vi "Read Config Settings from INI file.vi"(1 "Hardware Configuration":T1={"SEM X coil"="SEM-X", "SEM Y coil"="SEM-Y", "FIB X coil"="FIB/ao0", "FIB Y coil"="FIB/ao1", "FIB Detector"="FIB/ai1", "SEM Detectors"="Detectors", "Det min (V)"=-10.0, "Det max (V)"=10.0, "Eanable COM"=TRUE, "COM port"="COM1", "FIB Beam blank"="FIB/port0/line0", "FIB Ext Scan"="FIB/port0/line1", "Det. FIB-NI auto switch"="FIB/port0/line2", "Post #1up"="Log/ao0", "Post #1down"="Log/ao1", "Post #2up"="Log/ao2", "Post #2down"="Log/ao3", "Machine Type"=2, "FIB Faraday Cup"="FIB/ai3", "Configuration file"=path "D:/3D FIB-SEM Files/Feiss.ini", "SEM Max FOV (um)"=350.0, "Machine ID"="Jeiss6/Merlin-xxxx", "Save config file"=FALSE, "Temperature port"="COM3", "Brightness A"=35.0, "Contrast A"=28.0, "Detector B name"="ESB @ 600 V", "Brightness B"=30.0, "Contrast B"=38.0, "Logging Device"="Log"} {"Machine Type" items=["Feiss", "NVision", "Jeiss"]}) -> (8 "Hardware Configuration Out":T1={"SEM X coil"="SEM-X", "SEM Y coil"="SEM-Y", "FIB X coil"="FIB/ao0", "FIB Y coil"="FIB/ao1", "FIB Detector"="FIB/ai1", "SEM Detectors"="Detectors", "Det min (V)"=-10.0, "Det max (V)"=10.0, "Eanable COM"=TRUE, "COM port"="COM1", "FIB Beam blank"="FIB/port0/line0", "FIB Ext Scan"="FIB/port0/line1", "Det. FIB-NI auto switch"="FIB/port0/line2", "Post #1up"="Log/ao0", "Post #1down"="Log/ao1", "Post #2up"="Log/ao2", "Post #2down"="Log/ao3", "Machine Type"=2, "FIB Faraday Cup"="FIB/ai3", "Configuration file"=path "D:/3D FIB-SEM Files/Feiss.ini", "SEM Max FOV (um)"=350.0, "Machine ID"="Jeiss6/Merlin-xxxx", "Save config file"=FALSE, "Temperature port"="COM3", "Brightness A"=35.0, "Contrast A"=28.0, "Detector B name"="ESB @ 600 V", "Brightness B"=30.0, "Contrast B"=38.0, "Logging Device"="Log"} {"Machine Type" items=["Feiss", "NVision", "Jeiss"]})   [LabVIEW 2018]
panel:
  # "If you modify the Hardware Configuration Cluster in the Main Tclk.VI, you will probably have to drop new versions of those cluster controls into this VI to preserve and update the naming.\nIf you change the name of a cluster control, you will break the ability to look that control up in old .ini files because the changed key name will be different."
  # "Detector"
  # "Brightness & Contrast (%)"
  # "A       InLens"
  # "Detector"
  # "Brightness & Contrast (%)"
  # "A       InLens"
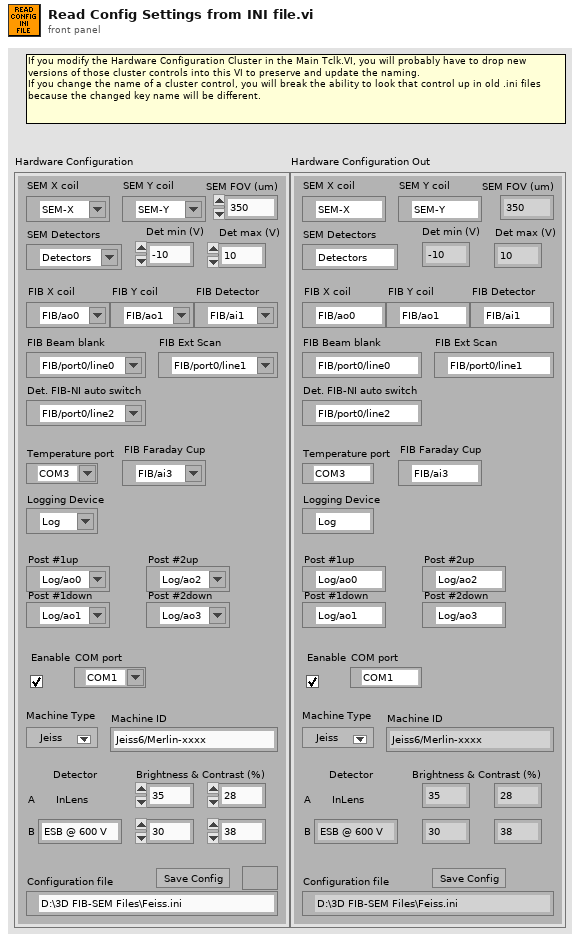
[diagram p1: front panel]
types:
  T1 = cluster{"SEM X coil":refnum<k15>, "SEM Y coil":refnum<k15>, "FIB X coil":tag, "FIB Y coil":tag, "FIB Detector":tag, "SEM Detectors":refnum<k15>, "Det min (V)":dbl, "Det max (V)":dbl, "Eanable COM":bool, "COM port":refnum<visa-resource-name>, "FIB Beam blank":tag, "FIB Ext Scan":tag, "Det. FIB-NI auto switch":tag, "Post #1up":tag, "Post #1down":tag, "Post #2up":tag, "Post #2down":tag, "Machine Type":u8, "FIB Faraday Cup":tag, "Configuration file":path, "SEM Max FOV (um)":sgl, "Machine ID":string, "Save config file":bool, "Temperature port":refnum<visa-resource-name>, "Brightness A":dbl, "Contrast A":dbl, "Detector B name":string, "Brightness B":dbl, "Contrast B":dbl, "Logging Device":tag}
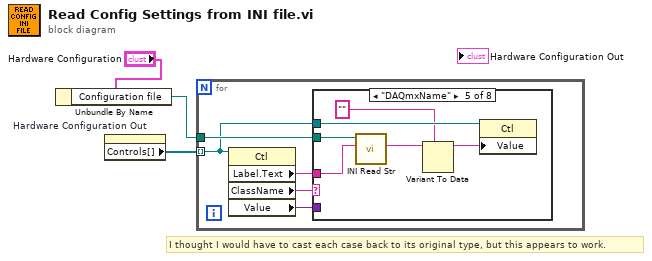
[diagram p0: block diagram]
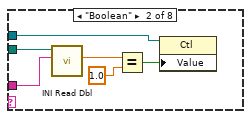
[diagram p3: hidden frame]
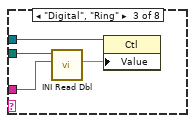
[diagram p4: hidden frame]
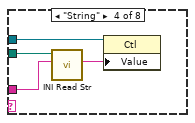
[diagram p5: hidden frame]
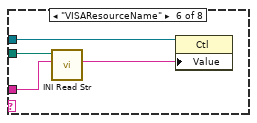
[diagram p6: hidden frame]
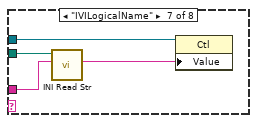
[diagram p7: hidden frame]
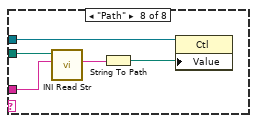
[diagram p8: hidden frame]
diagram:
  # "I thought I would have to cast each case back to its original type, but this appears to work."
  n1 = Unbundle By Name("Hardware Configuration") -> ("Configuration file"=w3:path)
  n2 = property on="Hardware Configuration Out" class="Clust (strict)"() -> ("Controls[]"=w2:refnum<vi>[])  [unwired: 2 in, 2 out]
  n3 = for {
    tunnel: w3 -> [w6]
    tunnel: w2 -> [w5] mode=indexing
    n4 = property class="Ctl"(reference=w5) -> ("Label.Text"=w7:string, "ClassName"=w8:string, "Value"=w4:variant)  [unwired: 1 in, 2 out]
    n5 = case shown="\"DAQmxName\"" w8 {
      tunnel: w7 -> [_ w14 w18 w20 w26 w30 w34 w39]
      tunnel: w6 -> [_ w13 w17 w21 w27 w31 w35 w40]
      tunnel: w5 -> [_ w12 w16 w22 w28 w32 w36 w41]
      tunnel: w4 -> [_ _ _ _ _ _ _ _]
      frame "False", Default {
      }
      frame "Boolean" {
        n6 = call "INI Read Dbl.vi"("Key Str"=w14, "configuration file path"=w13) -> ("Value Out"=w11:dbl)  [unwired: 7 in, 2 out]
        n7 = Equal?(x=w11, y=1.0) -> (x = y?=w9:bool)
        n8 = property class="Ctl"(reference=w12, "Value"=w9) -> ()  [unwired: 1 in, 2 out]
      }
      frame "Digital", "Ring" {
        n9 = call "INI Read Dbl.vi"("Key Str"=w18, "configuration file path"=w17) -> ("Value Out"=w15:dbl)  [unwired: 7 in, 2 out]
        n10 = property class="Ctl"(reference=w16, "Value"=w15) -> ()  [unwired: 1 in, 2 out]
      }
      frame "String" {
        n11 = call "INI Read Str.vi"("Key Str"=w20, "configuration file path"=w21) -> ("Str Out"=w19:string)  [unwired: 7 in, 2 out]
        n12 = property class="Ctl"(reference=w22, "Value"=w19) -> ()  [unwired: 1 in, 2 out]
      }
      frame "DAQmxName" {
        n13 = call "INI Read Str.vi"("Key Str"=w26, "configuration file path"=w27) -> ("Str Out"=w25:string)  [unwired: 7 in, 2 out]
        n14 = Variant To Data(type="", Variant=w25) -> (data=w24:string)  [unwired: 1 in, 1 out]
        n15 = property class="Ctl"(reference=w28, "Value"=w24) -> ()  [unwired: 1 in, 2 out]
      }
      frame "VISAResourceName" {
        n16 = call "INI Read Str.vi"("Key Str"=w30, "configuration file path"=w31) -> ("Str Out"=w29:string)  [unwired: 7 in, 2 out]
        n17 = property class="Ctl"(reference=w32, "Value"=w29) -> ()  [unwired: 1 in, 2 out]
      }
      frame "IVILogicalName" {
        n18 = call "INI Read Str.vi"("Key Str"=w34, "configuration file path"=w35) -> ("Str Out"=w33:string)  [unwired: 7 in, 2 out]
        n19 = property class="Ctl"(reference=w36, "Value"=w33) -> ()  [unwired: 1 in, 2 out]
      }
      frame "Path" {
        n20 = call "INI Read Str.vi"("Key Str"=w39, "configuration file path"=w40) -> ("Str Out"=w38:string)  [unwired: 7 in, 2 out]
        n21 = String To Path(string=w38) -> (path=w37:path)
        n22 = property class="Ctl"(reference=w41, "Value"=w37) -> ()  [unwired: 1 in, 2 out]
      }
    }
  }
